vi "MW_Display_Py_Open_Virtual.vi"(0 "Env path":path=path "D:/dev/Guy_Storage/.venv", 5 "Python version":string="3.12", 11 "error in":errorcluster) -> (4 "session out":refnum<k35>, 15 "error out":errorcluster)   [LabVIEW 2023]
uses:
  <vilib>/Python/Open Venv Python Session.vi
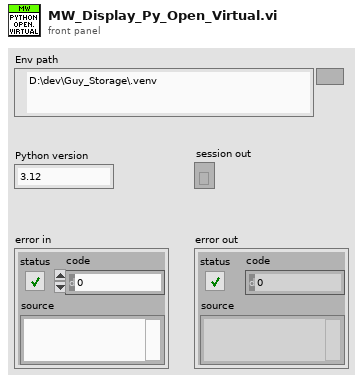
[diagram p1: front panel]
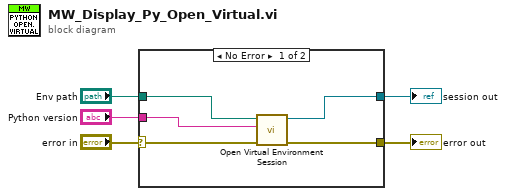
[diagram p0: block diagram]
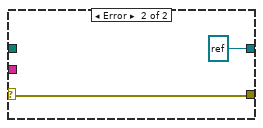
[diagram p2: hidden frame]
diagram:
  n1 = case shown="No Error" "error in" {
    selector: "error in" -> [w6 w12]
    tunnel: "Env path" -> [w10 _]
    tunnel: "Python version" -> [w9 _]
    tunnel: [w8 refnum<k35> refnum ("session out")] -> w3
    tunnel: [w7 w12] -> w2
    frame No Error {
      n2 = call-poly <vilib>:"Open Virtual Environment Session.vi"("error in (no error)"=w6, "Python version"=w9, "Env path"=w10) -> ("error out"=w7:errorcluster, "session out"=w8:refnum<k35>)  [unwired: 7 in]
    }
    frame Error {
    }
  }
  "session out" <- w3
  "error out" <- w2
